vi "signal spectrum analysis1.vi"() -> ()   [LabVIEW 2012]
uses:
  <vilib>/express/express analysis/Spectral/Block/exnSpectralBlock spectral measurements RMS poly.vi
  <vilib>/express/express analysis/Spectral/Block/exnSpectralBlock spectral measurements RMS DDT.vi
  <vilib>/express/express analysis/Spectral/XNode/ExpressSpectralMeasurementsBlockNode.xnode
panel:
  out "Filtered Signal":dynamicdata(graph)
  out "Waveform Graph 2":dynamicdata(graph)
  out "Waveform Graph":dynamicdata(graph)
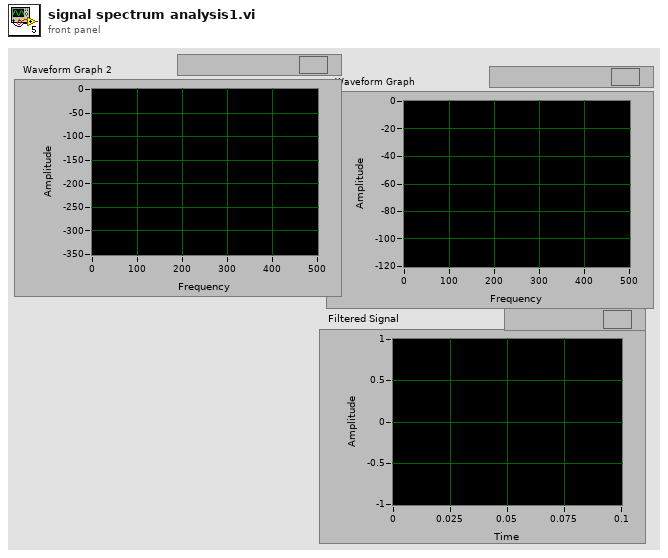
[diagram p1: front panel]
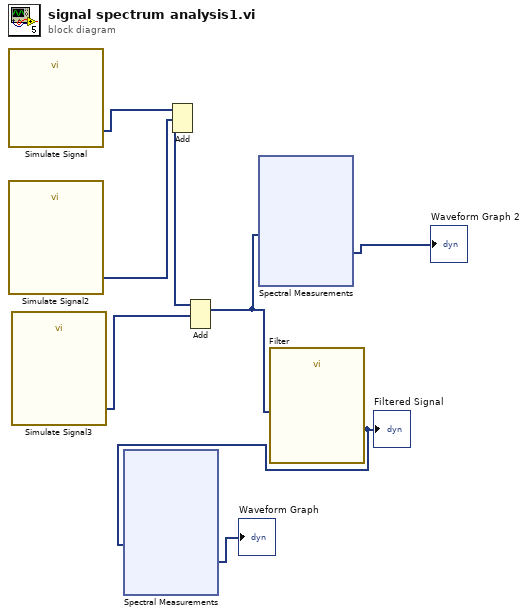
[diagram p0: block diagram]
diagram:
  n1 = call "Simulate Signal"() -> ("Sine"=w7:dynamicdata)  [unwired: 14 in, 1 out]
  n2 = call "Simulate Signal2"() -> ("Sine"=w6:dynamicdata)  [unwired: 14 in, 1 out]
  n3 = call "Simulate Signal3"() -> ("Sine"=w4:dynamicdata)  [unwired: 14 in, 1 out]
  n4 = Add(1:w6, 2:w7) -> (0:w5:dynamicdata)  [unwired: 1 in, 1 out]
  n5 = Add(1:w4, 2:w5) -> (0:w3:dynamicdata)  [unwired: 1 in, 1 out]
  n6 = xnode "Spectral Measurements"("Signals"=w3) -> ("FFT - (RMS)"=→"Waveform Graph 2":dynamicdata)  [unwired: 1 in, 2 out]
  n7 = call "Filter"("Signal"=w3) -> ("Filtered Signal"=w2:dynamicdata)  [unwired: 9 in, 1 out]
  "Filtered Signal" <- w2
  n8 = xnode "Spectral Measurements"("Signals"=w2) -> ("FFT - (RMS)"=→"Waveform Graph":dynamicdata)  [unwired: 1 in, 2 out]
